vi "CODMn报警信息转换.vi"(11 "报警簇":T1) -> (2 "CODMN报警信息备注":string, 3 "CODMN报警信息":string)   [LabVIEW 2016, in "斯坦道CODMn.lvlib"]
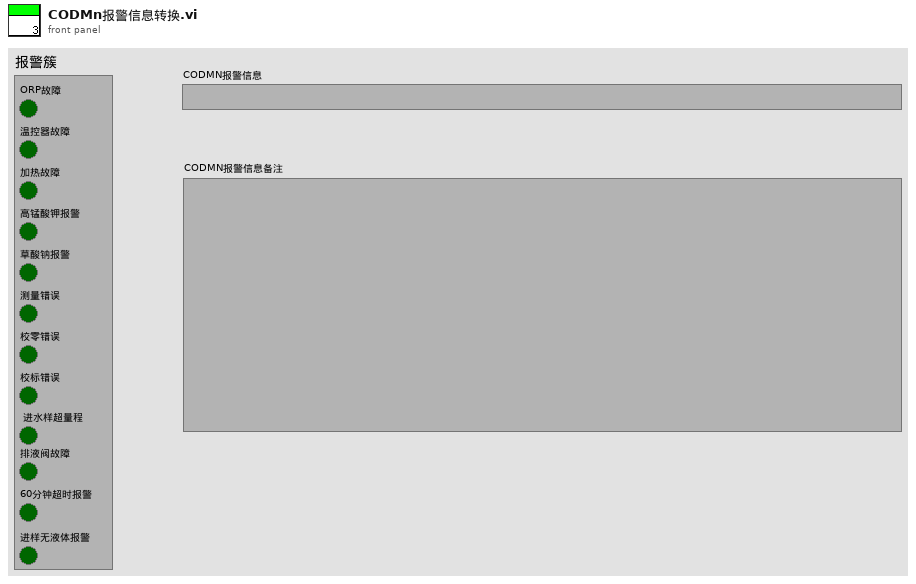
[diagram p1: front panel]
types:
  T1 = cluster{"ORP故障":bool, "温控器故障":bool, "加热故障":bool, "高锰酸钾报警":bool, "草酸钠报警":bool, "测量错误":bool, "校零错误":bool, "校标错误":bool, " 进水样超量程":bool, "排液阀故障":bool, "60分钟超时报警":bool, "进样无液体报警":bool}
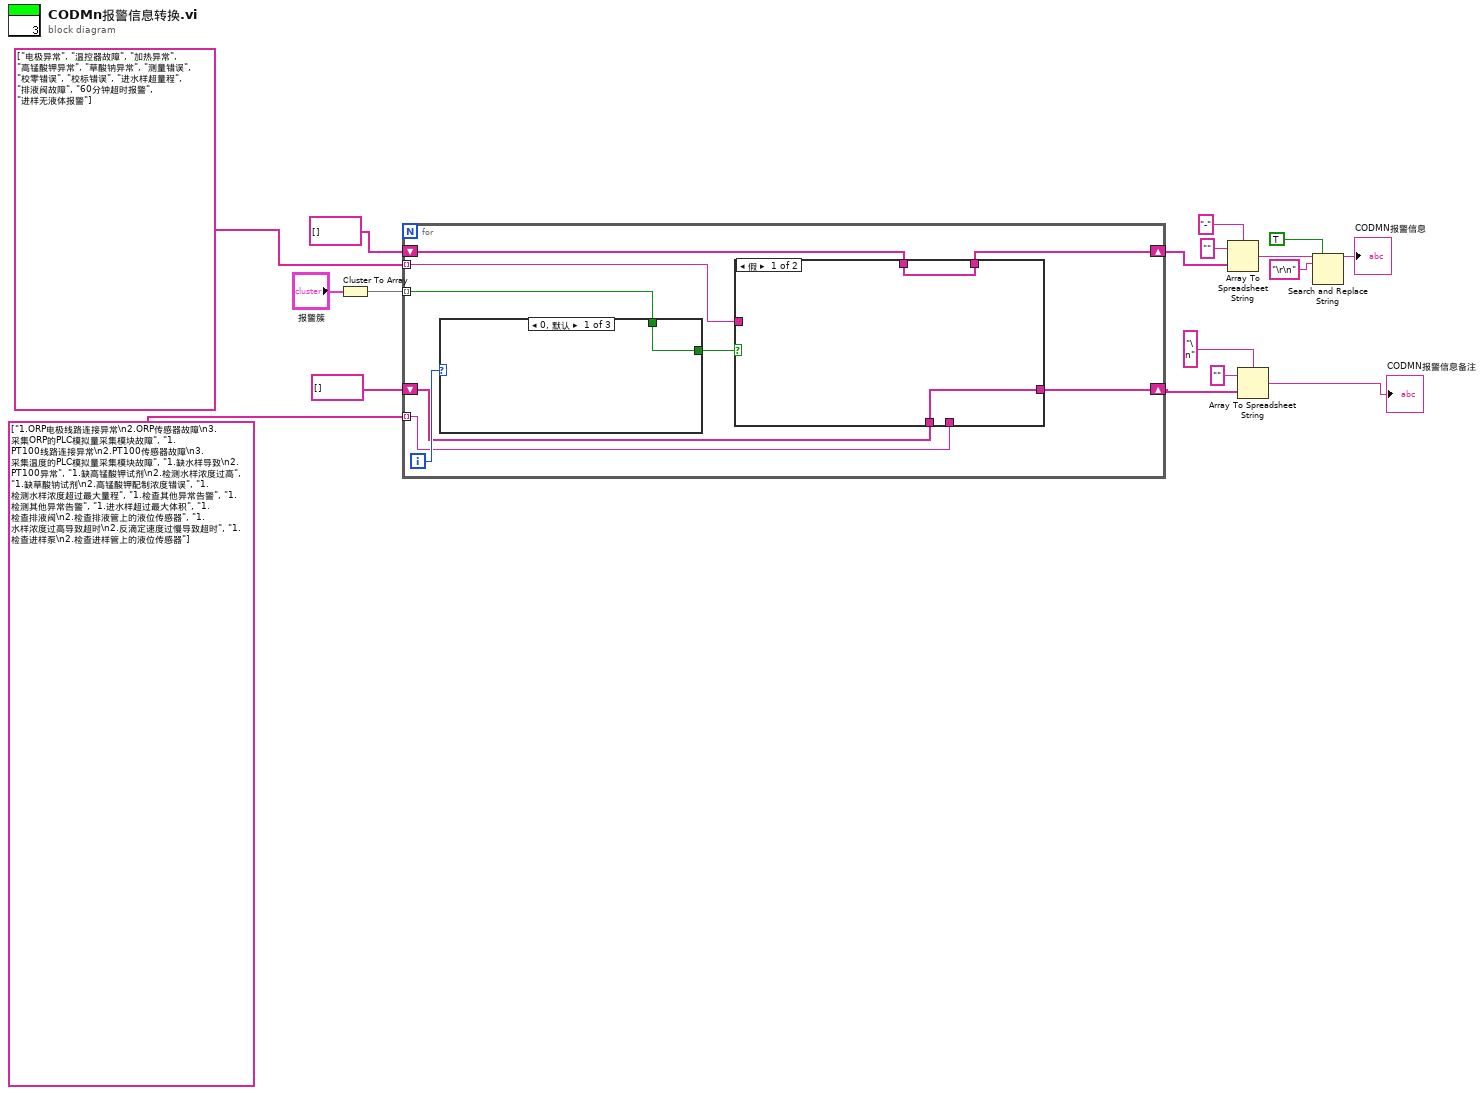
[diagram p0: block diagram]
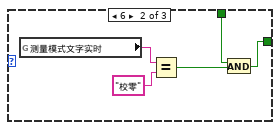
[diagram p2: hidden frame]
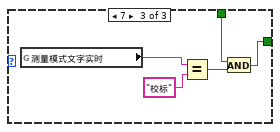
[diagram p3: hidden frame]
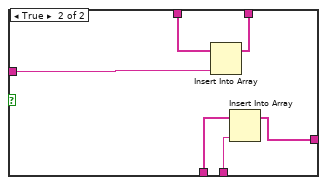
[diagram p4: hidden frame]
diagram:
  n1 = Cluster To Array(cluster="报警簇") -> (array=w10:bool[])
  n2 = for {
    tunnel: w10 -> [w25] mode=indexing
    shift-right: [w21] -> w5
    shift-left: string[] [] -> [w23]
    tunnel: string[] ["电极异常", "温控器故障", "加热异常", "高锰酸钾异常", "草酸钠异常", "测量错误", "校零错误", "校标错误", "进水样超量程", "排液阀故障", "60分钟超时报警", "进样无液体报警"] -> [w22] mode=indexing
    shift-right: [w18] -> w2
    shift-left: string[] [] -> [w20]
    tunnel: string[] ["1.ORP电极线路连接异常\n2.ORP传感器故障\n3.采集ORP的PLC模拟量采集模块故障", "1.PT100线路连接异常\n2.PT100传感器故障\n3.采集温度的PLC模拟量采集模块故障", "1.缺水样导致\n2.PT100异常", "1.缺高锰酸钾试剂\n2.检测水样浓度过高", "1.缺草酸钠试剂\n2.高锰酸钾配制浓度错误", "1.检测水样浓度超过最大量程", "1.检查其他异常告警", "1.检测其他异常告警", "1.进水样超过最大体积", "1.检查排液阀\n2.检查排液管上的液位传感器", "1.水样浓度过高导致超时\n2.反滴定速度过慢导致超时", "1.检查进样泵\n2.检查进样管上的液位传感器"] -> [w19] mode=indexing
    i -> [w26]
    n3 = case shown="0, 默认" w26 {
      tunnel: w25 -> [w27 w29 w34]
      tunnel: [w27 w28 w33] -> w24
      frame 0, Default {
      }
      frame 6 {
        n4 = global read "COD测量模式全局.vi" "测量模式文字实时"() -> (w31:string)
        n5 = Equal?(x=w31, y="校零" ("测量模式")) -> (x = y?=w30:bool)
        n6 = And(x=w29, y=w30) -> (x .and. y?=w28:bool)
      }
      frame 7 {
        n7 = global read "COD测量模式全局.vi" "测量模式文字实时"() -> (w36:string)
        n8 = Equal?(x=w36, y="校标" ("测量模式")) -> (x = y?=w35:bool)
        n9 = And(x=w34, y=w35) -> (x .and. y?=w33:bool)
      }
    }
    n10 = case shown="假" w24 {
      tunnel: w23 -> [w39 w45]
      tunnel: w22 -> [_ w44]
      tunnel: [w39 w43] -> w21
      tunnel: w20 -> [w38 w42]
      tunnel: w19 -> [_ w41]
      tunnel: [w38 w40] -> w18
      frame False {
      }
      frame True {
        n11 = Insert Into Array(array=w45, new element=w44) -> (w43:string[])  [unwired: 1 in]
        n12 = Insert Into Array(array=w42, new element=w41) -> (w40:string[])  [unwired: 1 in]
      }
    }
  }
  n13 = Array To Spreadsheet String(delimiter (Tab)="-" ("分隔符(Tab)"), array=w5, 3:"" ("格式字符串")) -> (spreadsheet string=w13:string)
  n14 = Array To Spreadsheet String(delimiter (Tab)="\n" ("分隔符(Tab)"), array=w2, 3:"" ("格式字符串")) -> (spreadsheet string=→"CODMN报警信息备注":string)
  n15 = Search and Replace String(replace all?=TRUE ("替换全部？(F)"), input string=w13, search string="\r\n" ("搜索字符串")) -> (result string=→"CODMN报警信息":string)  [unwired: 5 in, 3 out]
